vi "LakeShore 370 Set Power.vi"(0 "Heater Power (W)":sgl, 1 "Lakeshore GPIB Address":refnum<visa-resource-name>) -> ()   [LabVIEW 2019]
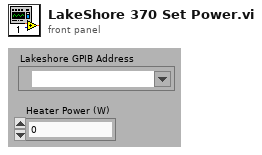
[diagram p1: front panel]
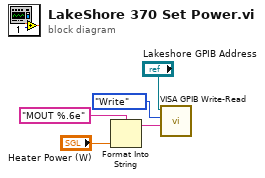
[diagram p0: block diagram]
diagram:
  n1 = Format Into String(format string="MOUT %.6e" ("initial string"), "Heater Power (W)") -> (resulting string=w2:string)  [unwired: 2 in, 1 out]
  n2 = call "VISA GPIB Write-Read.vi"("Command"=w2, "Action"=enum16{"Write", "Read", "Write & Read"}."Write", "VISA resource name"="Lakeshore GPIB Address") -> ()  [unwired: 5 in, 4 out]
